vi "Core Extraction.vi"(5 "Dimension1":i32, 7 "Dimension2":i32, 9 "Offset Dim 2":i32, 10 "Offset Dim 1":i32, 11 "Core extraction size":i32) -> (2 "Core rectangle":T1, 3 "Code Dims":cluster{i32, i32, i32, i32})   [LabVIEW 2020]
panel:
  out "dim2_length":i32
  out "dim2_start":i32
  out "dim1_length":i32
  out "dim1_start":i32
  out "output variable 6":dbl
  out "output variable 5":dbl
  out "output variable 4":dbl
  out "output variable 3":dbl
  out "output variable 2":i32
  out "output variable":i32
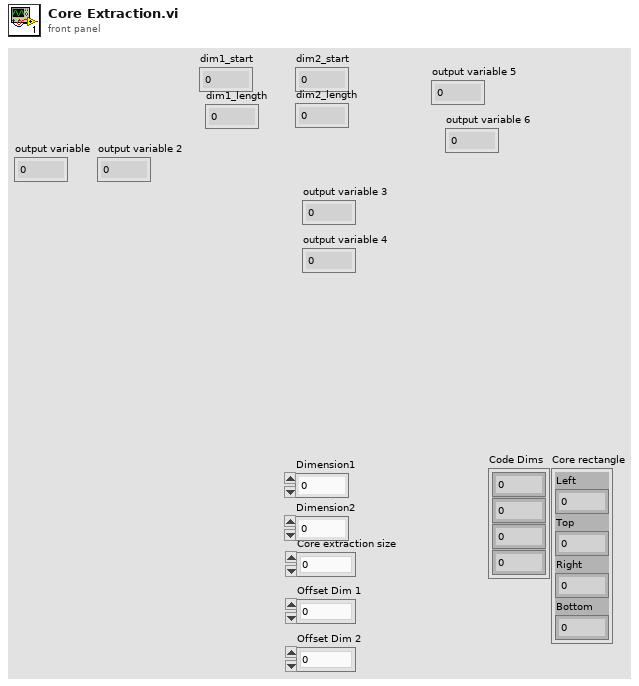
[diagram p1: front panel]
types:
  T1 = cluster{"Left":i32, "Top":i32, "Right":i32, "Bottom":i32}
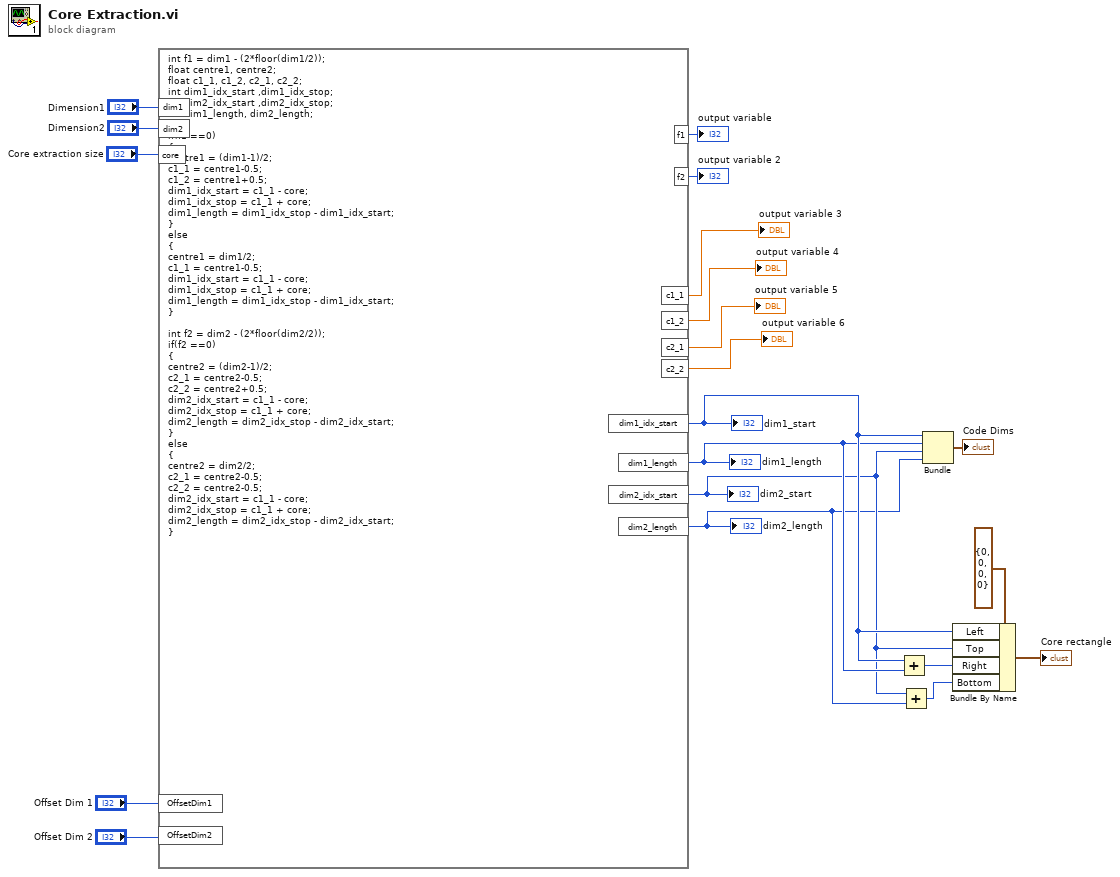
[diagram p0: block diagram]
diagram:
  n1 = formula code="int f1 = dim1 - (2*floor(dim1/2));\nfloat centre1, centre2;\nfloat c1_1, c1_2, c2_1, c2_2;\nint dim1_idx_start ,dim1_idx_stop;\nint dim2_idx_start ,dim2_idx_stop;\nint dim1_length, dim2_length;\n\nif(f1 ==0)\n{\ncentre1 = (dim1-1)/2;\nc1_1 = centre1-0.5;\nc1_2 = centre1+0.5;\ndim1_idx_start = c1_1 - core;\ndim1_idx_stop = c1_1 + core;\ndim1_length = dim1_idx_stop - dim1_idx_start;\n}\nelse\n{\ncentre1 = dim1/2;\nc1_1 = centre1-0.5;\ndim1_idx_start = c1_1 - core;\ndim1_idx_stop = c1_1 + core;\ndim1_length = dim1_idx_stop - dim1_idx_start;\n}\n\nint f2 = dim2 - (2*floor(dim2/2));\nif(f2 ==0)\n{\ncentre2 = (dim2-1)/2;\nc2_1 = centre2-0.5;\nc2_2 = centre2+0.5;\ndim2_idx_start = c1_1 - core;\ndim2_idx_stop = c1_1 + core;\ndim2_length = dim2_idx_stop - dim2_idx_start;\n}\nelse\n{\ncentre2 = dim2/2;\nc2_1 = centre2-0.5; \nc2_2 = centre2-0.5;\ndim2_idx_start = c1_1 - core;\ndim2_idx_stop = c1_1 + core;\ndim2_length = dim2_idx_stop - dim2_idx_start;\n}"("dim1"="Dimension1", "dim2"="Dimension2", "core"="Core extraction size", "OffsetDim1"="Offset Dim 1", "OffsetDim2"="Offset Dim 2") -> ("f1"=→"output variable":i32, "f2"=→"output variable 2":i32, "c1_1"=→"output variable 3":dbl, "c1_2"=→"output variable 4":dbl, "c2_1"=→"output variable 5":dbl, "c2_2"=→"output variable 6":dbl, "dim1_idx_start"=w9:i32, "dim1_length"=w8:i32, "dim2_idx_start"=w6:i32, "dim2_length"=w5:i32)
  "dim1_start" <- w9
  "dim1_length" <- w8
  "dim2_start" <- w6
  "dim2_length" <- w5
  n2 = Add(x=w9, y=w8) -> (x+y=w7:i32)
  n3 = Add(x=w6, y=w5) -> (x+y=w4:i32)
  n4 = Bundle(w9, w8, w6, w5) -> (→"Code Dims":cluster{i32, i32, i32, i32})  [unwired: 1 in]
  n5 = Bundle By Name(cluster=T1 {"Left"=0, "Top"=0, "Right"=0, "Bottom"=0} ("Rectangle"), "Left"=w9, "Top"=w6, "Right"=w7, "Bottom"=w4) -> (→"Core rectangle":T1)
